vi "Keithley 2182_6221.vi"() -> ()   [LabVIEW 2017]
doc: "Stores specified measurements in buffer and reads the contents of the buffer as well as its statistics."
uses:
  <instrlib>/Keithley 622x LV 2009/Configure/Source/Typedefs/KE622x -- Current Range.ctl
  <instrlib>/Keithley 622x LV 2009/Configure/Source/Typedefs/KE622x -- Current Ranges.ctl
  <instrlib>/Keithley 622x LV 2009/Typedefs/KE622x -- On Off Control.ctl
  <instrlib>/Keithley 622x LV 2009/Utility/Typedefs/KE622x -- Instrument Type.ctl
  <instrlib>/Keithley 622x LV 2009/Configure/Output/Typedefs/KE6221 -- Output Response.ctl
  <instrlib>/Keithley 622x LV 2009/Configure/Source/Typedefs/KE622x -- Current Level.ctl
  <instrlib>/Keithley 622x LV 2009/Configure/Source/Typedefs/KE622x -- Voltage Limit.ctl
  <vilib>/Analysis/baseanly.llb/Mean (DBL).vi
  <instrlib>/Keithley 2182/Keithley 2182.lvlib
  <vilib>/Analysis/NI_AALBase.lvlib
  <instrlib>/Keithley 622x LV 2009/Keithley 622x.lvlib
panel:
  out "output cluster":T1={"mean"=0.0, "seconds since 1Jan1904"=timestamp(3592862696.5384784 s since 1904-01-01)}
  in  "Save Data":bool=TRUE
  in  "Tab Control":enum32{"File"}(tab)
  in  "Filename":string="Voltmeter"
  out "file path":path=path "C:/Users/aspitarl/Google Drive/NETL/Labview/Learn/TDMS test/2017-11-06/Voltmeter.tdms"
  in  "base path":path=path "C:/Users/aspitarl/Google Drive/NETL/Labview/Learn/TDMS test"
  in  "Output State":T2
  in  "Turn Off Output If Voltage Limit?":bool=TRUE
  out "error out":errorcluster={"status"=TRUE, "code"=-1073807346, "source"="VISA Open in Keithley 622x.lvlib:Initialize.vi->Keithley 2182 Custom_add6221.vi"}
  out "Voltage Limit?":bool
  out "Interlock Tripped?":bool
  in  "Voltage Limit (V)":T3=10.0 min=0.1 max=105.0 step=0.01 format="%.2p"
  in  "Current Level (A)":T4=0.001 min=-0.105 max=0.105 format="%.4p"
  in  "Output Response":T5=enum."Slow"
  in  "Instrument Type":T6=enum."KE6221"
  in  "Analog Filter State":T2
  in  "Current Range In":T7={"Auto Range?"=TRUE, "Man / Selected\nRange"=enum."2nA"}
  in  "Check For SCPI Errors? (T)":bool=TRUE
  in  "VISA resource name 2":refnum<visa-resource-name>="TCPIP0::192.168.000.002::1394::SOCKET"
  out "XY Graph":cluster{timestamp[], dbl[]}(graph)={[timestamp(3592862694.8584785 s since 1904-01-01), timestamp(3592862694.8724785 s since 1904-01-01), timestamp(3592862694.8814783 s since 1904-01-01), timestamp(3592862694.8924785 s since 1904-01-01), timestamp(3592862694.9044785 s since 1904-01-01), timestamp(3592862694.9164786 s since 1904-01-01), timestamp(3592862694.9304786 s since 1904-01-01), timestamp(3592862694.942478 s since 1904-01-01), timestamp(3592862694.9564786 s since 1904-01-01), timestamp(3592862694.9664783 s since 1904-01-01), timestamp(3592862694.9784784 s since 1904-01-01), timestamp(3592862694.988478 s since 1904-01-01), timestamp(3592862694.9954786 s since 1904-01-01), timestamp(3592862695.0054784 s since 1904-01-01), timestamp(3592862695.0134783 s since 1904-01-01), timestamp(3592862695.0194783 s since 1904-01-01), timestamp(3592862695.0304785 s since 1904-01-01), timestamp(3592862695.0434785 s since 1904-01-01), timestamp(3592862695.0564785 s since 1904-01-01), timestamp(3592862695.0714784 s since 1904-01-01), timestamp(3592862695.086478 s since 1904-01-01), timestamp(3592862695.1044784 s since 1904-01-01), timestamp(3592862695.1224785 s since 1904-01-01), timestamp(3592862695.1414785 s since 1904-01-01), timestamp(3592862695.1534786 s since 1904-01-01), timestamp(3592862695.165478 s since 1904-01-01), timestamp(3592862695.1774783 s since 1904-01-01), timestamp(3592862695.1904783 s since 1904-01-01), timestamp(3592862695.2024784 s since 1904-01-01), timestamp(3592862695.2194786 s since 1904-01-01), timestamp(3592862695.2294784 s since 1904-01-01), timestamp(3592862695.2414784 s since 1904-01-01), timestamp(3592862695.2524786 s since 1904-01-01), timestamp(3592862695.2624784 s since 1904-01-01), timestamp(3592862695.2874784 s since 1904-01-01), timestamp(3592862695.2994785 s since 1904-01-01), timestamp(3592862695.310478 s since 1904-01-01), timestamp(3592862695.3214784 s since 1904-01-01), timestamp(3592862695.3394785 s since 1904-01-01), timestamp(3592862695.3514786 s since 1904-01-01), timestamp(3592862695.3614783 s since 1904-01-01), timestamp(3592862695.369478 s since 1904-01-01), timestamp(3592862695.3804784 s since 1904-01-01), timestamp(3592862695.3904786 s since 1904-01-01), timestamp(3592862695.3974786 s since 1904-01-01), timestamp(3592862695.409478 s since 1904-01-01), timestamp(3592862695.4214783 s since 1904-01-01), timestamp(3592862695.4384785 s since 1904-01-01), timestamp(3592862695.4644785 s since 1904-01-01), timestamp(3592862695.4784784 s since 1904-01-01), timestamp(3592862695.4914784 s since 1904-01-01), timestamp(3592862695.5044785 s since 1904-01-01), timestamp(3592862695.521478 s since 1904-01-01), timestamp(3592862695.5364785 s since 1904-01-01), timestamp(3592862695.5534782 s since 1904-01-01), timestamp(3592862695.5664783 s since 1904-01-01), timestamp(3592862695.5774784 s since 1904-01-01), timestamp(3592862695.5984783 s since 1904-01-01), timestamp(3592862695.6164784 s since 1904-01-01), timestamp(3592862695.6444783 s since 1904-01-01), timestamp(3592862695.6584783 s since 1904-01-01), timestamp(3592862695.6734786 s since 1904-01-01), timestamp(3592862695.6894784 s since 1904-01-01), timestamp(3592862695.7044783 s since 1904-01-01), timestamp(3592862695.7324786 s since 1904-01-01), timestamp(3592862695.7424784 s since 1904-01-01), timestamp(3592862695.7544785 s since 1904-01-01), timestamp(3592862695.7664785 s since 1904-01-01), timestamp(3592862695.7914786 s since 1904-01-01), timestamp(3592862695.8094783 s since 1904-01-01), timestamp(3592862695.8214784 s since 1904-01-01), timestamp(3592862695.8334785 s since 1904-01-01), timestamp(3592862695.8584785 s since 1904-01-01), timestamp(3592862695.8734784 s since 1904-01-01), timestamp(3592862695.8784785 s since 1904-01-01), timestamp(3592862695.8864784 s since 1904-01-01), timestamp(3592862695.8924785 s since 1904-01-01), timestamp(3592862695.9004784 s since 1904-01-01), timestamp(3592862695.9084783 s since 1904-01-01), timestamp(3592862695.9174786 s since 1904-01-01), timestamp(3592862695.9234786 s since 1904-01-01), timestamp(3592862695.9284782 s since 1904-01-01), timestamp(3592862695.9344783 s since 1904-01-01), timestamp(3592862695.9414783 s since 1904-01-01), timestamp(3592862695.9494786 s since 1904-01-01), timestamp(3592862695.955478 s since 1904-01-01), timestamp(3592862695.9644785 s since 1904-01-01), timestamp(3592862695.9734783 s since 1904-01-01), timestamp(3592862695.981478 s since 1904-01-01), timestamp(3592862695.9894786 s since 1904-01-01), timestamp(3592862695.9964786 s since 1904-01-01), timestamp(3592862696.0044785 s since 1904-01-01), timestamp(3592862696.0134783 s since 1904-01-01), timestamp(3592862696.0194783 s since 1904-01-01), timestamp(3592862696.027478 s since 1904-01-01), timestamp(3592862696.0364785 s since 1904-01-01), timestamp(3592862696.0434785 s since 1904-01-01), timestamp(3592862696.0494785 s since 1904-01-01), timestamp(3592862696.0574784 s since 1904-01-01), timestamp(3592862696.0634785 s since 1904-01-01), timestamp(3592862696.0694785 s since 1904-01-01), timestamp(3592862696.0844784 s since 1904-01-01), timestamp(3592862696.0964785 s since 1904-01-01), timestamp(3592862696.1054783 s since 1904-01-01), timestamp(3592862696.1114783 s since 1904-01-01), timestamp(3592862696.1204786 s since 1904-01-01), timestamp(3592862696.1284785 s since 1904-01-01), timestamp(3592862696.1374784 s since 1904-01-01), timestamp(3592862696.146478 s since 1904-01-01), timestamp(3592862696.1544785 s since 1904-01-01), timestamp(3592862696.1704783 s since 1904-01-01), timestamp(3592862696.1824784 s since 1904-01-01), timestamp(3592862696.1914783 s since 1904-01-01), timestamp(3592862696.1994786 s since 1904-01-01), timestamp(3592862696.2084785 s since 1904-01-01), timestamp(3592862696.2154784 s since 1904-01-01), timestamp(3592862696.2244782 s since 1904-01-01), timestamp(3592862696.238478 s since 1904-01-01), timestamp(3592862696.2594786 s since 1904-01-01), timestamp(3592862696.2684784 s since 1904-01-01), timestamp(3592862696.2764783 s since 1904-01-01), timestamp(3592862696.284478 s since 1904-01-01), timestamp(3592862696.2894783 s since 1904-01-01), timestamp(3592862696.2984786 s since 1904-01-01), timestamp(3592862696.3054786 s since 1904-01-01), timestamp(3592862696.317478 s since 1904-01-01), timestamp(3592862696.336478 s since 1904-01-01), timestamp(3592862696.3454785 s since 1904-01-01), timestamp(3592862696.3544784 s since 1904-01-01), timestamp(3592862696.3624783 s since 1904-01-01), timestamp(3592862696.369478 s since 1904-01-01), timestamp(3592862696.3754783 s since 1904-01-01), timestamp(3592862696.382478 s since 1904-01-01), timestamp(3592862696.3934784 s since 1904-01-01), timestamp(3592862696.3994784 s since 1904-01-01), timestamp(3592862696.4084783 s since 1904-01-01), timestamp(3592862696.4174786 s since 1904-01-01), timestamp(3592862696.4274783 s since 1904-01-01), timestamp(3592862696.4334784 s since 1904-01-01), timestamp(3592862696.4404783 s since 1904-01-01), timestamp(3592862696.455478 s since 1904-01-01), timestamp(3592862696.4744782 s since 1904-01-01), timestamp(3592862696.4834785 s since 1904-01-01), timestamp(3592862696.4894786 s since 1904-01-01), timestamp(3592862696.4984784 s since 1904-01-01), timestamp(3592862696.507478 s since 1904-01-01), timestamp(3592862696.514478 s since 1904-01-01), timestamp(3592862696.5224786 s since 1904-01-01), timestamp(3592862696.5304785 s since 1904-01-01), timestamp(3592862696.5384784 s since 1904-01-01)], [0.0, 0.0, 0.0, 0.0, 0.0, 0.0, 0.0, 0.0, 0.0, 0.0, 0.0, 0.0, 0.0, 0.0, 0.0, 0.0, 0.0, 0.0, 0.0, 0.0, 0.0, 0.0, 0.0, 0.0, 0.0, 0.0, 0.0, 0.0, 0.0, 0.0, 0.0, 0.0, 0.0, 0.0, 0.0, 0.0, 0.0, 0.0, 0.0, 0.0, 0.0, 0.0, 0.0, 0.0, 0.0, 0.0, 0.0, 0.0, 0.0, 0.0, 0.0, 0.0, 0.0, 0.0, 0.0, 0.0, 0.0, 0.0, 0.0, 0.0, 0.0, 0.0, 0.0, 0.0, 0.0, 0.0, 0.0, 0.0, 0.0, 0.0, 0.0, 0.0, 0.0, 0.0, 0.0, 0.0, 0.0, 0.0, 0.0, 0.0, 0.0, 0.0, 0.0, 0.0, 0.0, 0.0, 0.0, 0.0, 0.0, 0.0, 0.0, 0.0, 0.0, 0.0, 0.0, 0.0, 0.0, 0.0, 0.0, 0.0, 0.0, 0.0, 0.0, 0.0, 0.0, 0.0, 0.0, 0.0, 0.0, 0.0, 0.0, 0.0, 0.0, 0.0, 0.0, 0.0, 0.0, 0.0, 0.0, 0.0, 0.0, 0.0, 0.0, 0.0, 0.0, 0.0, 0.0, 0.0, 0.0, 0.0, 0.0, 0.0, 0.0, 0.0, 0.0, 0.0, 0.0, 0.0, 0.0, 0.0, 0.0, 0.0, 0.0, 0.0, 0.0, 0.0, 0.0, 0.0, 0.0, 0.0]}
  out "Measurements Metadata":T9(array[cluster])
  out "Measurements":dbl[](array[numeric])
  in  "Stop":bool
  in  "Selected Calculation Settings":enum32{"Linear Settings", "Percent Settings"}(tab)
  in  "Offset Value (0)":dbl
  in  "Scale Factor (1)":dbl=1.0
  in  "Units (MX)":string="MX"
  in  "Use Input Signal as Target Value (F: Disable)":bool
  in  "Target Value (1)":dbl=1.0
  in  "Selected Measurement Settings":enum32{"Voltage Settings", "Temp Settings"}(tab)
  in  "Voltage Resolution (8)":i32=8
  in  "Range Value (10)":dbl=10.0
  in  "Autorange (T: Enable)":bool=TRUE
  in  "Sensor (1: Internal)":i32(ring)=1 items=["Thermocouple", "Internal"]
  in  "Reference Junction Type (0: Internal)":i32(ring) items=["Internal", "Simulated"]
  in  "Simulated Reference Temp (23 C)":dbl=23.0
  in  "Thermocouple Type (0: J)":i32(ring) items=["J", "K", "T", "E", "R", "S", "B", "N"]
  in  "Temperature Resolution (6)":i32=6
  in  "Unit (0: Celsius)":i32(ring) items=["Celsius", "Fahrenheit", "Kelvin"]
  in  "Math Calculation (0: Linear)":i32(ring) items=["Linear", "Percent"]
  in  "Measurement (0: Voltage Channel 1)":i32(ring) items=["Voltage Channel 1", "Voltage Channel 2", "Temperature Channel 1", "Temperature Channel 2"]
  in  "Integration Rate Units (0: Line Cycles)":i32(ring) items=["Line Cycles", "Seconds"]
  in  "Integration Rate (5)":dbl=5.0
  in  "Buffer Source (0: None)":i32(ring)=1 items=["None", "Measurements", "Math Calculation"]
  in  "Buffer Size (10)":i32=10
  in  "VISA resource name":refnum<visa-resource-name>="COM4"
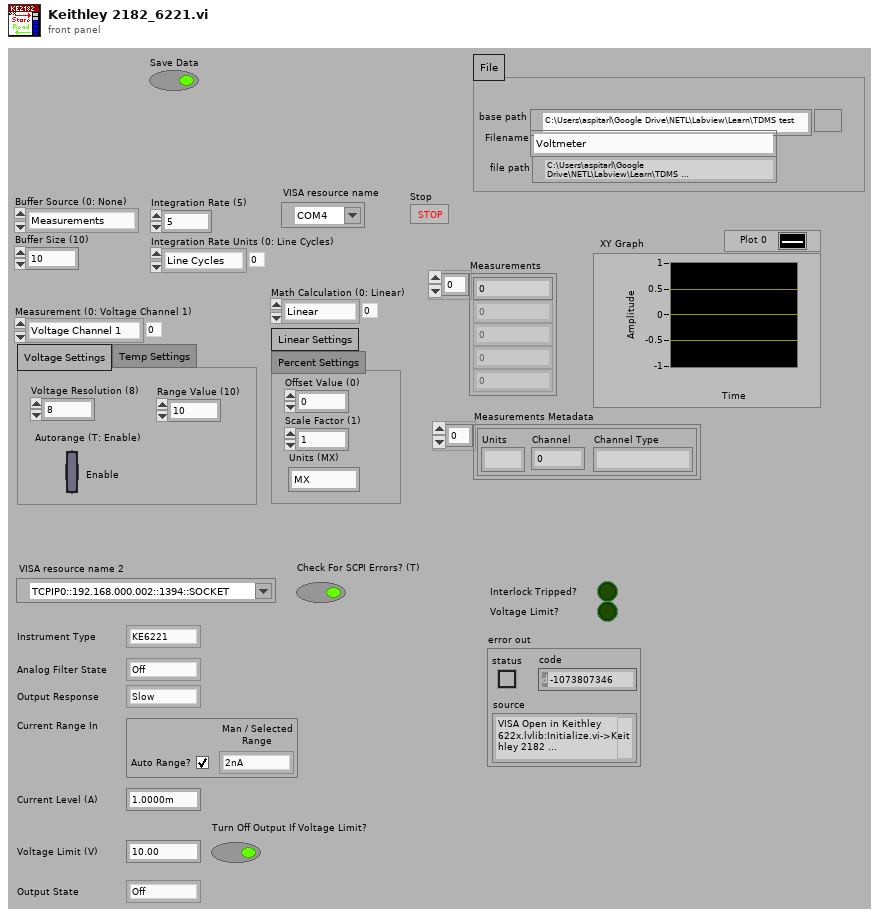
[diagram p1: front panel]
types:
  T1 = cluster{"mean":dbl, "seconds since 1Jan1904":timestamp}
  T2 = typedef "Keithley 622x.lvlib/KE622x -- On Off Control.ctl" = enum16{"Off", "On"}
  T3 = typedef "Keithley 622x.lvlib/KE622x -- Voltage Limit.ctl" = dbl
  T4 = typedef "Keithley 622x.lvlib/KE622x -- Current Level.ctl" = dbl
  T5 = typedef "Keithley 622x.lvlib/KE6221 -- Output Response.ctl" = enum16{"Fast", "Slow"}
  T6 = typedef "Keithley 622x.lvlib/KE622x -- Instrument Type.ctl" = enum16{"KE6220", "KE6221"}
  T7 = typedef "Keithley 622x.lvlib/KE622x -- Current Range.ctl" = cluster{"Auto Range?":bool, "Man / Selected\nRange":T8}
  T8 = typedef "Keithley 622x.lvlib/KE622x -- Current Ranges.ctl" = enum16{"2nA", "20nA", "200nA", "2uA", "20uA", "200uA", "2mA", "20mA", "100mA"}
  T9 = cluster{"Units":string, "Channel":i32, "Channel Type":string}[]
  T10 = enum16{"open", "open or create", "create or replace", "create", "open (read-only)"}
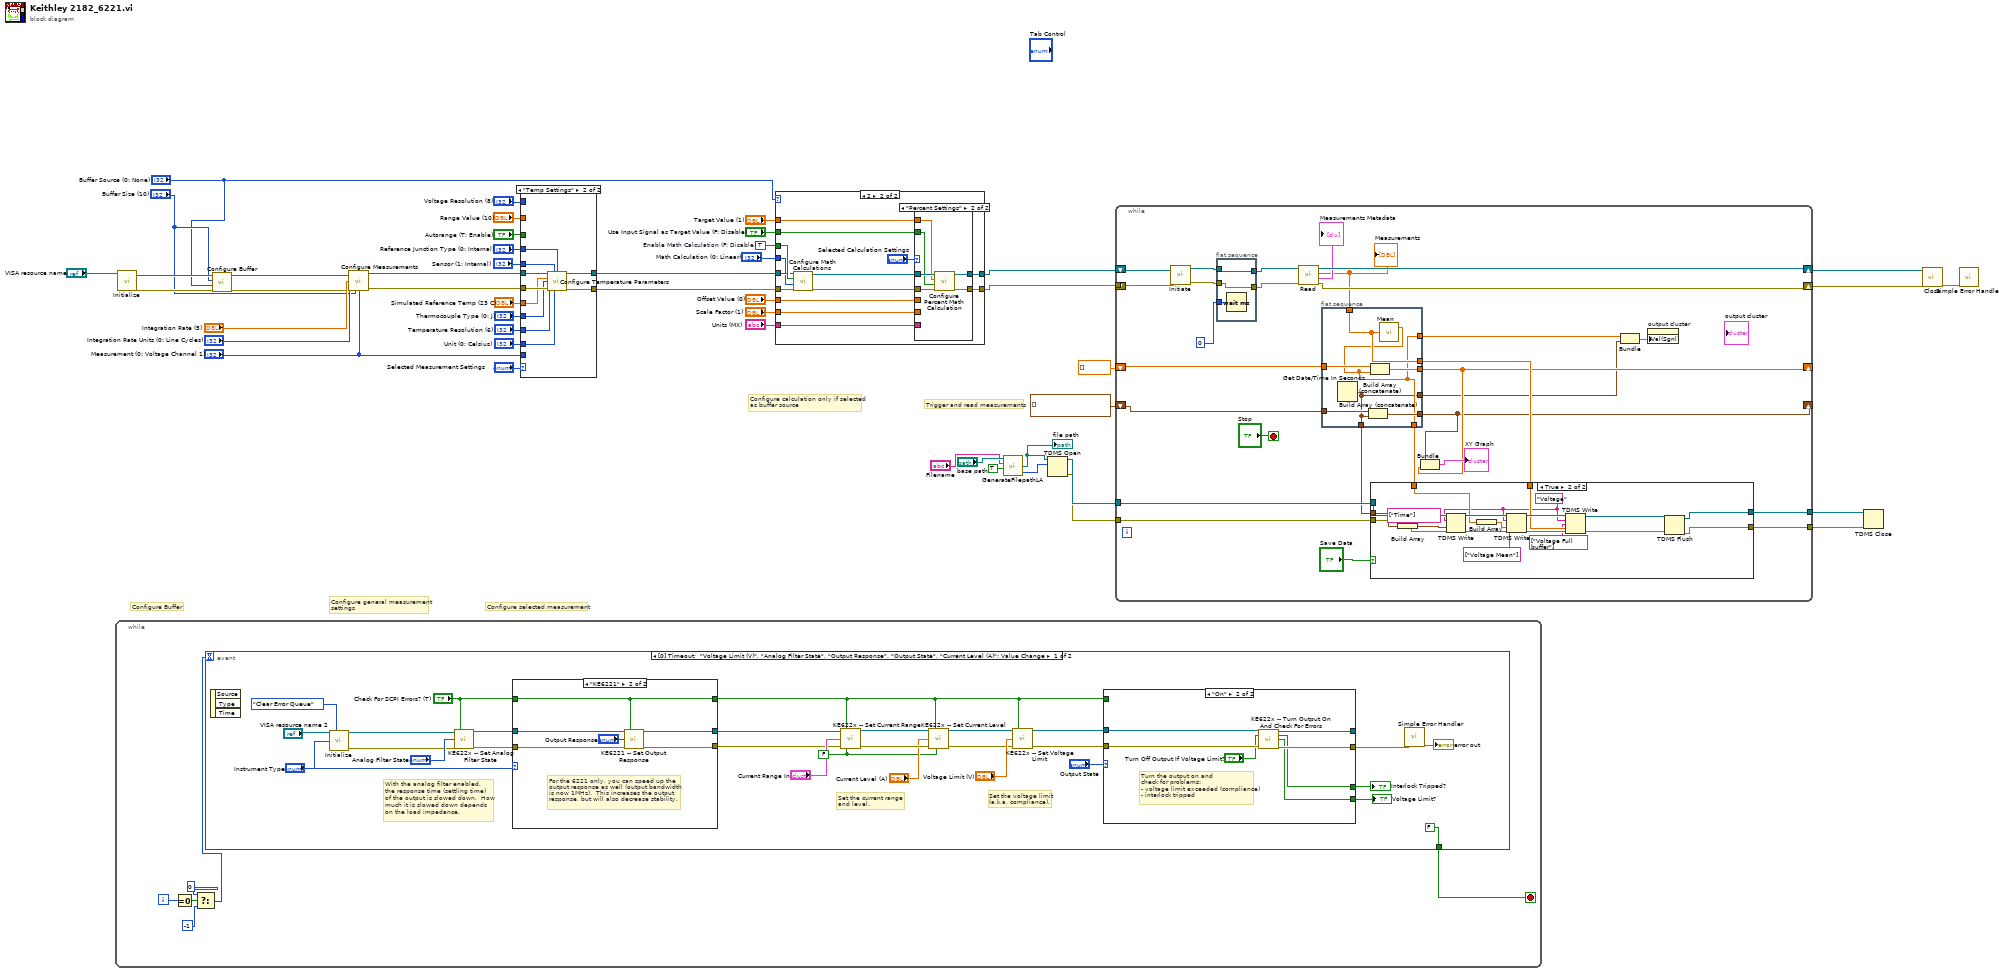
[diagram p0: block diagram]
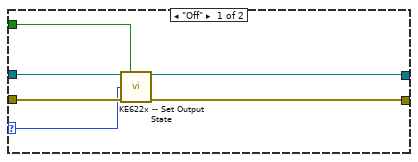
[diagram p2: hidden frame]
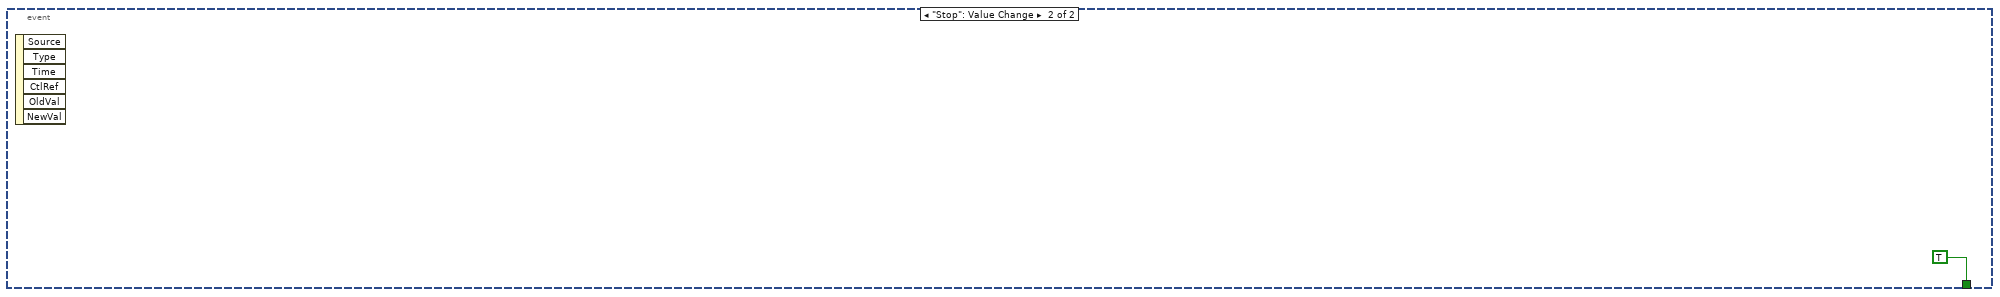
[diagram p4: hidden frame]
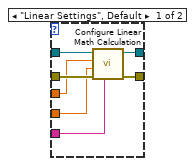
[diagram p7: hidden frame]
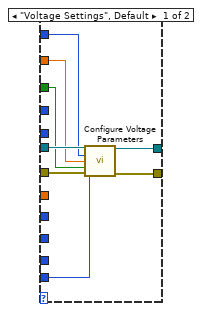
[diagram p8: hidden frame]
diagram:
  w33 = TRUE  # Enable Math Calculation (F: Disable)
  # "Trigger and read measurements"
  # "Configure general measurement\nsettings"
  # "Configure Buffer"
  # "Configure calculation only if selected\nas buffer source"
  # "Configure selected measurement"
  n1 = while {
    i -> [w52]
    stop <- w53 stop-if-true
    n2 = Equal To 0?(x=w52) -> (x = 0?=w51:bool)
    n3 = Select(t=0, s=w51, f=-1) -> (s? t:f=w48:i32)
    n4 = event shown="[0] Timeout;  \"Voltage Limit (V)\", \"Analog Filter State\", \"Output Response\", \"Output State\", \"Current Level (A)\": Value Change" {
      selector: _ -> [_ _]
      dyn-events: _ -> [_ _]
      timeout: w48 -> [_ _]
      tunnel: [FALSE TRUE] -> w53
      event Timeout; Value Change {
        w71 = FALSE ("Read Back Set Values? (T)")
        # "Set the voltage limit\n(a.k.a. compliance)."
        # "Set the current range\nand level."
        # "With the analog filter enabled,\nthe response time (settling time)\nof the output is slowed down.  How\nmuch it is slowed down depends\non the load impedance."
        n5 = event-data() -> ()  [unwired: 1 in, 3 out]
        n6 = call <instrlib>:"Initialize.vi"("VISA resource name"="VISA resource name 2", "Error Queue Option"=enum16{"Clear Error Queue", "Error Query"}."Clear Error Queue", "Instrument Type"="Instrument Type") -> ("VISA resource name out"=w57:refnum<visa-resource-name>, "error out"=w56:errorcluster)  [unwired: 11 in]
        n7 = call <instrlib>:"KE622x -- Set Analog Filter State.vi"("Resource In"=w57, "Check For SCPI Errors? (T)"="Check For SCPI Errors? (T)", "Analog Filter State"="Analog Filter State", "error in (no error)"=w56) -> ("Resource Out (dupl)"=w79:refnum<visa-resource-name>, "error out"=w78:errorcluster)  [unwired: 10 in]
        n8 = case shown="\"KE6221\"" "Instrument Type" {
          tunnel: w79 -> [w96 w103]
          tunnel: w78 -> [w95 w101]
          tunnel: [w96 w100] -> w75
          tunnel: "Check For SCPI Errors? (T)" -> [w97 w99]
          tunnel: [w97 w99] -> w64
          tunnel: [w95 w98] -> w76
          frame "KE6220" {
          }
          frame "KE6221" {
            # "For the 6221 only, you can speed up the\noutput response as well (output bandwidth\nis now 1MHz).  This increases the output\nresponse, but will also decrease stability."
            n9 = call <instrlib>:"KE6221 -- Set Output Response.vi"("Resource In"=w103, "Check For SCPI Errors? (T)"=w99, "KE6221 Output Response"="Output Response", "error in (no error)"=w101) -> ("Resource Out (dupl)"=w100:refnum<visa-resource-name>, "error out"=w98:errorcluster)  [unwired: 10 in]
          }
        }
        n10 = call <instrlib>:"KE622x -- Set Current Range.vi"("Resource In"=w75, "Check For SCPI Errors? (T)"=w64, "Current Range In"="Current Range In", "error in (no error)"=w76, "Read Back Set Values? (T)"=w71) -> ("Resource Out (dupl)"=w74:refnum<visa-resource-name>, "error out"=w73:errorcluster)  [unwired: 8 in, 1 out]
        n11 = call <instrlib>:"KE622x -- Set Current Level.vi"("Resource In"=w74, "Check For SCPI Errors? (T)"=w64, "Current Level (A) In"="Current Level (A)", "error in (no error)"=w73, "Read Back Set Value? (T)"=w71) -> ("Resource Out (dupl)"=w69:refnum<visa-resource-name>, "error out"=w68:errorcluster)  [unwired: 8 in, 1 out]
        n12 = call <instrlib>:"KE622x -- Set Voltage Limit.vi"("Resource In"=w69, "Check For SCPI Errors? (T)"=w64, "Voltage Limit (V)"="Voltage Limit (V)", "error in (no error)"=w68) -> ("Resource Out (dupl)"=w67:refnum<visa-resource-name>, "error out"=w66:errorcluster)  [unwired: 10 in]
        n13 = case shown="\"On\"" "Output State" {
          selector: "Output State" -> [w85 _]
          tunnel: w67 -> [w87 w94]
          tunnel: w66 -> [w86 w93]
          tunnel: [w83 w91] -> w54
          tunnel: w64 -> [w84 _]
          tunnel: [_ w90] -> w63
          tunnel: [_ w89] -> w62
          tunnel: [w82 w88] -> _
          frame "Off" {
            n14 = call <instrlib>:"KE622x -- Set Output State.vi"("Resource In"=w87, "Check For SCPI Errors? (T)"=w84, "Output State"=w85, "error in (no error)"=w86) -> ("Resource Out (dupl)"=w82:refnum<visa-resource-name>, "error out"=w83:errorcluster)  [unwired: 10 in]
          }
          frame "On" {
            # "Turn the output on and\ncheck for problems:\n- voltage limit exceeded (compliance)\n- interlock tripped"
            n15 = call <instrlib>:"KE622x -- Turn Output On And Check For Errors.vi"("Resource In"=w94, "Turn Off Output If Compliance?"="Turn Off Output If Voltage Limit?", "error in (no error)"=w93) -> ("Resource Out (dupl)"=w88:refnum<visa-resource-name>, "Interlock Tripped?"=w90:bool, "Compliance?"=w89:bool, "error out"=w91:errorcluster)  [unwired: 9 in]
          }
        }
        "Interlock Tripped?" <- w63
        "Voltage Limit?" <- w62
        n16 = call <vilib>:"Simple Error Handler.vi"("error in (no error)"=w54) -> ("error out"=→"error out":errorcluster)  [unwired: 4 in, 4 out]
      }
      event "Stop": Value Change {
        n17 = event-data() -> ()  [unwired: 1 in, 6 out]
      }
    }
  }
  n18 = call <instrlib>:"Initialize.vi"("VISA resource name"="VISA resource name") -> ("error out"=w14:errorcluster, "VISA resource name out"=w15:refnum<visa-resource-name>)  [unwired: 9 in]
  n19 = call <instrlib>:"Configure Buffer.vi"("error in (no error)"=w14, "Buffer Source (0: None)"="Buffer Source (0: None)", "Buffer Size (2)"="Buffer Size (10)", "VISA resource name"=w15) -> ("error out"=w17:errorcluster, "VISA resource name out"=w16:refnum<visa-resource-name>)  [unwired: 6 in]
  n20 = call <instrlib>:"Configure Measurements.vi"("VISA resource name"=w16, "Measurement (0: Voltage Channel 1)"="Measurement (0: Voltage Channel 1)", "Integration Rate (5)"="Integration Rate (5)", "Integration Rate Units (0: Line Cycles)"="Integration Rate Units (0: Line Cycles)", "error in (no error)"=w17, "Sample Count (1)"="Buffer Size (10)") -> ("VISA resource name out"=w40:refnum<visa-resource-name>, "error out"=w41:errorcluster)  [unwired: 8 in]
  n21 = case shown="\"Temp Settings\"" "Selected Measurement Settings" {
    tunnel: "Voltage Resolution (8)" -> [w106 _]
    tunnel: "Range Value (10)" -> [w107 _]
    tunnel: "Autorange (T: Enable)" -> [w108 _]
    tunnel: w41 -> [w112 w122]
    tunnel: w40 -> [w111 w121]
    tunnel: [w110 w120] -> w30
    tunnel: [w109 w119] -> w31
    tunnel: "Unit (0: Celsius)" -> [_ w118]
    tunnel: "Temperature Resolution (6)" -> [_ w117]
    tunnel: "Thermocouple Type (0: J)" -> [_ w116]
    tunnel: "Simulated Reference Temp (23 C)" -> [_ w115]
    tunnel: "Sensor (1: Internal)" -> [_ w114]
    tunnel: "Reference Junction Type (0: Internal)" -> [_ w113]
    tunnel: "Measurement (0: Voltage Channel 1)" -> [w105 _]
    frame "Voltage Settings", Default {
      n22 = call <instrlib>:"Configure Voltage Parameters.vi"("VISA resource name"=w111, "Measurement (1: Voltage Channel 1)"=w105, "Voltage Resolution (8)"=w106, "Range Value (12)"=w107, "Autorange (T: Enable)"=w108, "error in (no error)"=w112) -> ("VISA resource name out"=w110:refnum<visa-resource-name>, "error out"=w109:errorcluster)  [unwired: 8 in]
    }
    frame "Temp Settings" {
      n23 = call <instrlib>:"Configure Temperature Parameters.vi"("VISA resource name"=w121, "Sensor (0: Thermocouple)"=w114, "Reference Junction Type (0: Internal)"=w113, "Simulated Reference Temp (23 C)"=w115, "Thermocouple Type (0: J)"=w116, "Temperature Resolution (6)"=w117, "error in (no error)"=w122, "Unit (0: Celsius)"=w118) -> ("VISA resource name out"=w120:refnum<visa-resource-name>, "error out"=w119:errorcluster)  [unwired: 6 in]
    }
  }
  n24 = case shown="2" "Buffer Source (0: None)" {
    tunnel: w33 -> [_ w138]
    tunnel: "Math Calculation (0: Linear)" -> [_ w135]
    tunnel: w31 -> [w124 w137]
    tunnel: w30 -> [w123 w136]
    tunnel: "Use Input Signal as Target Value (F: Disable)" -> [_ w134]
    tunnel: "Target Value (1)" -> [_ w133]
    tunnel: "Offset Value (0)" -> [_ w130]
    tunnel: "Scale Factor (1)" -> [_ w129]
    tunnel: "Units (MX)" -> [_ w128]
    tunnel: [w124 w127] -> w22
    tunnel: [w123 w126] -> w21
    frame 0, Default {
    }
    frame 2 {
      n25 = call <instrlib>:"Configure Math Calculations.vi"("error in (no error)"=w137, "Math Calculation (0: Linear)"=w135, "Enable Math Calculation (F: Disable)"=w138, "VISA resource name"=w136) -> ("error out"=w132:errorcluster, "VISA resource name out"=w131:refnum<visa-resource-name>)  [unwired: 6 in]
      n26 = case shown="\"Percent Settings\"" "Selected Calculation Settings" {
        tunnel: w134 -> [_ w147]
        tunnel: w133 -> [_ w146]
        tunnel: w132 -> [w145 w148]
        tunnel: w131 -> [w144 w149]
        tunnel: w130 -> [w143 _]
        tunnel: w129 -> [w142 _]
        tunnel: w128 -> [w141 _]
        tunnel: [w140 w151] -> w127
        tunnel: [w139 w150] -> w126
        frame "Linear Settings", Default {
          n27 = call <instrlib>:"Configure Linear Math Calculation.vi"("Units (MX)"=w141, "error in (no error)"=w145, "Offset Value (0)"=w142, "Scale Factor (1)"=w143, "VISA resource name"=w144) -> ("error out"=w140:errorcluster, "VISA resource name out"=w139:refnum<visa-resource-name>)  [unwired: 5 in]
        }
        frame "Percent Settings" {
          n28 = call <instrlib>:"Configure Percent Math Calculation.vi"("error in (no error)"=w148, "Use Input Signal as Target Value (F: Disable)"=w147, "Target Value (1)"=w146, "VISA resource name"=w149) -> ("error out"=w151:errorcluster, "VISA resource name out"=w150:refnum<visa-resource-name>)  [unwired: 6 in]
        }
      }
    }
  }
  n29 = call "GenerateFilepathLA.vi"("Auto Date folder"=TRUE, "Filename"="Filename", "base path"="base path") -> ("operation (0:open)"=w6:T10, "file path"=w7:path)  [unwired: 1 in, 1 out]
  "file path" <- w7
  n30 = TDMS Open(10:w6, 11:w7) -> (0:w4:errorcluster, 3:w5:refnum<k34>)  [unwired: 5 in]
  n31 = while {
    shift-right: [w171] -> w20
    shift-left: w21 -> [w175]
    tunnel: w22 -> [w174]
    shift-right: [w170] -> w18
    shift-left: _ -> [_]
    shift-right: [w156] -> _
    shift-left: dbl[] [] -> [w167]
    shift-right: [w155] -> _
    shift-left: timestamp[] [] -> [w166]
    tunnel: w5 -> [w164]
    tunnel: w4 -> [w163]
    tunnel: [w158] -> w3
    tunnel: [w157] -> w2
    stop <- "Stop" stop-if-true
    n32 = call <instrlib>:"Initiate.vi"("error in (no error)"=w174, "VISA resource name"=w175) -> ("error out"=w177:errorcluster, "VISA resource name out"=w176:refnum<visa-resource-name>)  [unwired: 8 in]
    n33 = flat-sequence {
      tunnel: u32 0 ("milliseconds to wait") -> [w210]
      tunnel: [w209] -> w172
      tunnel: [w208] -> w173
      tunnel: w177 -> [w209]
      tunnel: w176 -> [w208]
      frame #0 {
        n34 = Wait (ms)(milliseconds to wait=w210) -> ()  [unwired: 1 out]
      }
    }
    n35 = call <instrlib>:"Read.vi"("error in (no error)"=w172, "VISA resource name"=w173) -> ("error out"=w170:errorcluster, "Measurements Metadata"=→"Measurements Metadata":T9, "Measurements"=w168:dbl[], "VISA resource name out"=w171:refnum<visa-resource-name>)  [unwired: 6 in]
    "Measurements" <- w168
    n36 = flat-sequence {
      tunnel: w168 -> [w203]
      tunnel: [w207] -> w156
      tunnel: w167 -> [w206]
      tunnel: [w205] -> w155
      tunnel: w166 -> [w204]
      tunnel: [w201] -> w161
      tunnel: [w202] -> w160
      tunnel: [w203] -> w159
      tunnel: [w202] -> w154
      tunnel: [w201] -> w153
      frame #0 {
        n37 = Get Date/Time In Seconds() -> (seconds since 1Jan1904=w201:timestamp)
        n38 = Build Array (concatenate)(w204, w201) -> (w205:timestamp[])
        n39 = call-poly <vilib>:"Mean.vi"("X"=w203) -> ("mean"=w202:dbl)  [unwired: 1 out]
        n40 = Build Array (concatenate)(w206, w202) -> (w207:dbl[])
      }
    }
    n41 = case shown="True" "Save Data" {
      tunnel: w164 -> [w181 w200]
      tunnel: w163 -> [w180 w199]
      tunnel: w161 -> [_ w198]
      tunnel: w160 -> [_ w193]
      tunnel: w159 -> [_ w188]
      tunnel: [w181 w183] -> w158
      tunnel: [w180 w182] -> w157
      frame False {
      }
      frame True {
        w186 = "Voltage" ("group name in (Untitled)")
        n42 = Build Array(w198) -> (w197:timestamp[])
        n43 = TDMS Write(0:w200, 5:w186, 7:string[] ["Time"] ("channel name(s) in (Untitled)"), 9:w197, 11:w199) -> (4:w195:refnum<k34>, 15:w194:errorcluster)  [unwired: 1 in, 2 out]
        n44 = Build Array(w193) -> (w192:dbl[])
        n45 = TDMS Write(0:w195, 5:w186, 7:string[] ["Voltage Mean"] ("channel name(s) in (Untitled)"), 9:w192, 11:w194) -> (4:w190:refnum<k34>, 15:w189:errorcluster)  [unwired: 1 in, 2 out]
        n46 = TDMS Write(0:w190, 5:w186, 7:string[] ["Voltage Full buffer"] ("channel name(s) in (Untitled)"), 9:w188, 11:w189) -> (4:w185:refnum<k34>, 15:w184:errorcluster)  [unwired: 1 in, 2 out]
        n47 = TDMS Flush(4:w184, 7:w185) -> (0:w182:errorcluster, 3:w183:refnum<k34>)
      }
    }
    n48 = Bundle(w155, w156) -> (→"XY Graph":cluster{timestamp[], dbl[]})  [unwired: 1 in]
    n49 = Bundle("mean"=w154, "seconds since 1Jan1904"=w153) -> (w152:T1)  [unwired: 1 in]
    n50 = property on="output cluster" class="Clust (strict)"("Val(Sgnl)"=w152) -> ()  [unwired: 2 in, 2 out]
  }
  n51 = TDMS Close(8:w2, 11:w3) -> ()  [unwired: 2 out]
  n52 = call <instrlib>:"Close.vi"("error in (no error)"=w18, "VISA resource name"=w20) -> ("error out"=w19:errorcluster)  [unwired: 9 in]
  n53 = call <vilib>:"Simple Error Handler.vi"("error in (no error)"=w19) -> ()  [unwired: 4 in, 5 out]
